vi "Read Response.vi"(8 "error in (no error)":errorcluster, 11 "API Message in":refnum<class "API Message.lvclass">) -> (0 "error out":errorcluster, 2 "Response.lvclass":refnum<class "Response.lvclass">, 3 "API Message out":refnum<class "API Message.lvclass">)   [LabVIEW 2023, in "API Message.lvclass"]
uses:
  API Message.lvclass
  Response/Response.lvclass
  API Message.lvclass/API Message.ctl
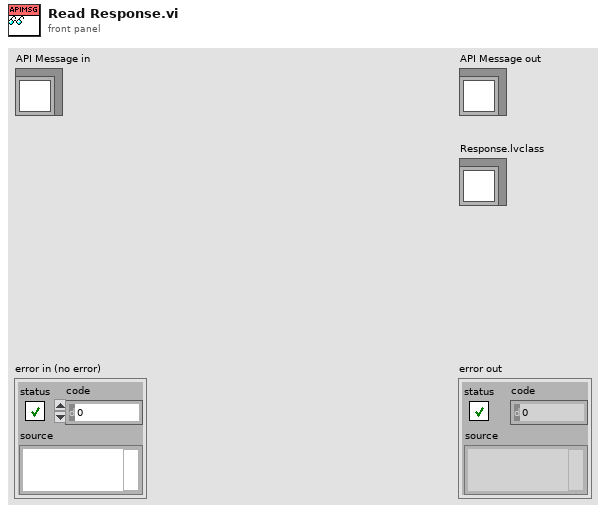
[diagram p1: front panel]
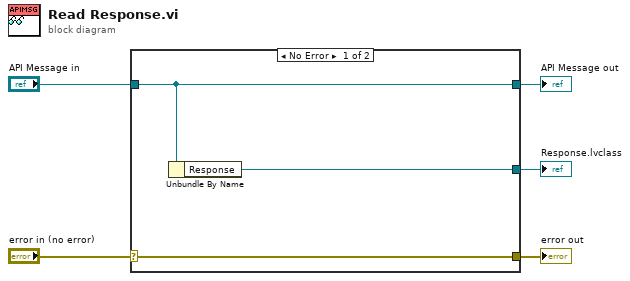
[diagram p0: block diagram]
diagram:
  n1 = case shown="No Error" "error in (no error)" {
    selector: "error in (no error)" -> [w8 w9]
    tunnel: [w8 w9] -> w4
    tunnel: [w7 w10] -> w2
    tunnel: "API Message in" -> [w7 w10]
    tunnel: [w6 _] -> w1
    frame No Error {
      n2 = Unbundle By Name(w7) -> ("Response"=w6:refnum<class "Response.lvclass">)
    }
    frame Error {
    }
  }
  "error out" <- w4
  "API Message out" <- w2
  "Response.lvclass" <- w1
